vi "RT main.vi"   [LabVIEW 2015]
uses:
  Setpoints.ctl
  <vilib>/Utility/error.llb/Error Cluster From Error Code.vi
  <vilib>/rvi/errors/niLvFpgaAdjustHostInterfaceError.vi
  <vilib>/FPGAPlugInAG/Dynamic/niLvFpga_Close_Dynamic.vi
  <vilib>/FPGAPlugInAG/cRIO-9118/niLvFpga_Open_cRIO-9118.vi
  <vilib>/rvi/interface/common/dynamic/niFpgaDynamicAddResources.vi
  <vilib>/FPGAPlugInAG/Dynamic/niLvFpga_Run_Dynamic.vi
  <vilib>/rvi/interface/nirviReadWriteControl/nirviReadWriteControl.xnode
  <vilib>/rvi/interface/nirviCloseFPGA/nirviCloseFPGA.xnode
  <vilib>/rvi/interface/nirviOpenFPGA/nirviOpenFPGA.xnode
  FPGA Bitfiles/TanqueQuadruplo_FPGATarget_FPGAmain_2eouoVfTWZU.lvbitx
  FPGA main.vi
  <vilib>/rvi/interface/nirviMethod/nirviMethod.xnode
  NiFpgaLv.dll
  <vilib>/rvi/interface/Simulation/niFpgaSimulationCallBeginRW.vi
types:
  T1 = typedef "Setpoints.ctl" = cluster{"Bomba 1":fxp<+/-,20,5>, "Bomba 2":fxp<+/-,20,5>, "Solenoide 1":bool, "Solenoide 2":bool, "Solenoide 3":bool, "Solenoide 4":bool, "Valvula proporcional 2":fxp<+/-,20,5>, "Valvula proporcional 1":fxp<+/-,20,5>}
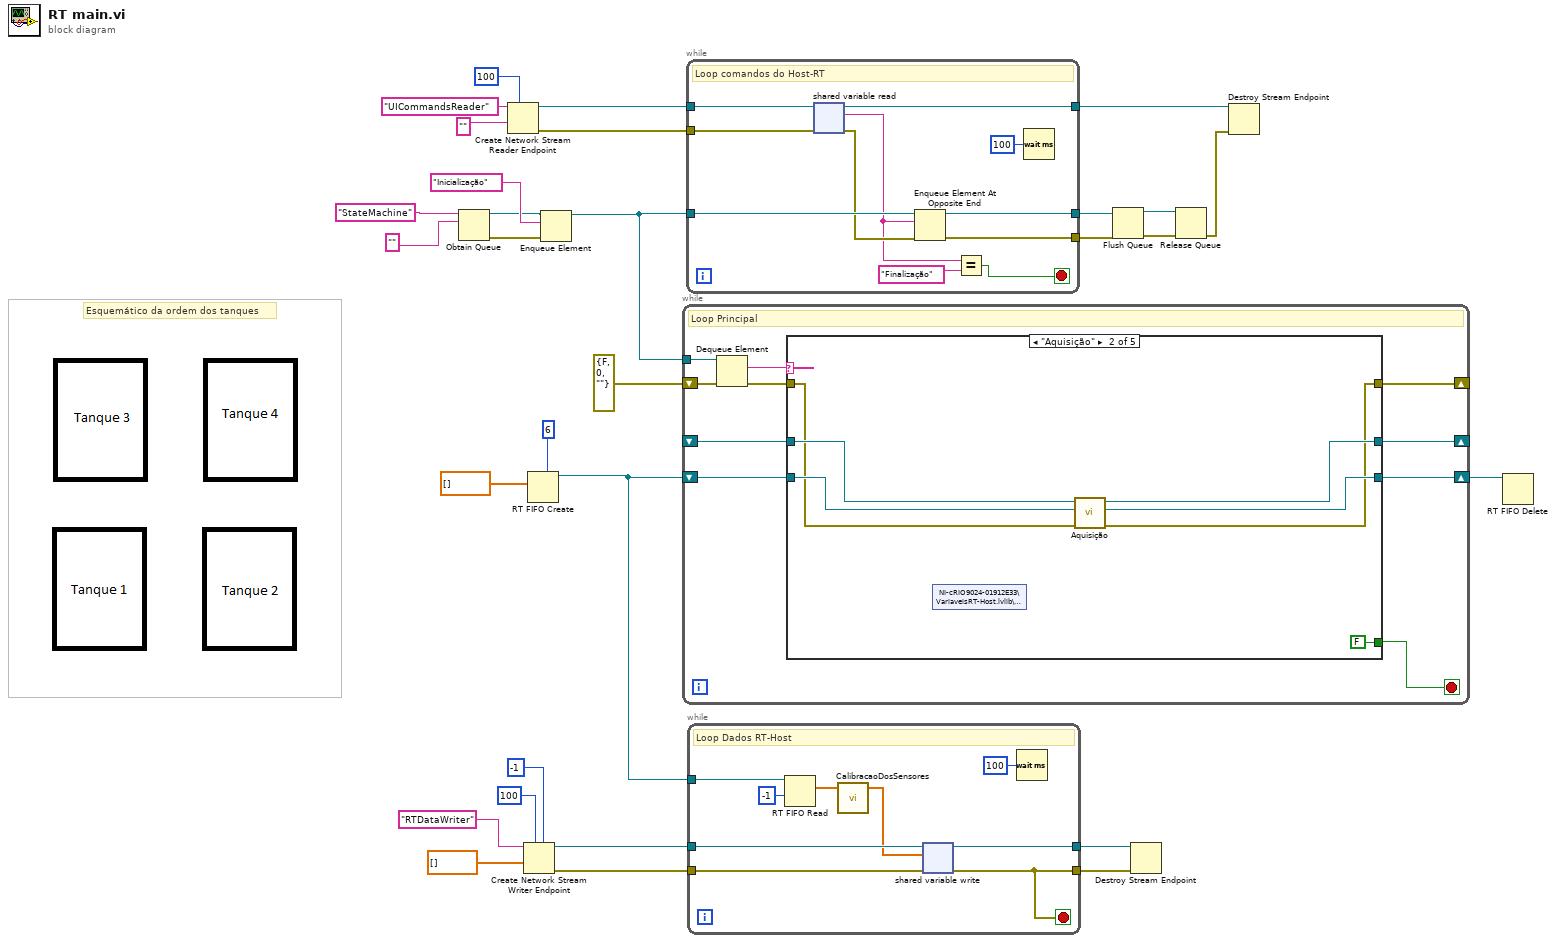
[diagram p0: block diagram]
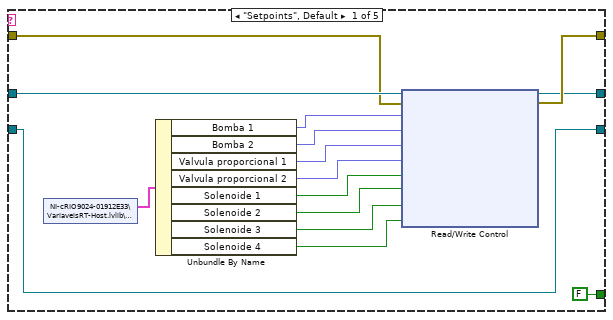
[diagram p2: hidden frame]
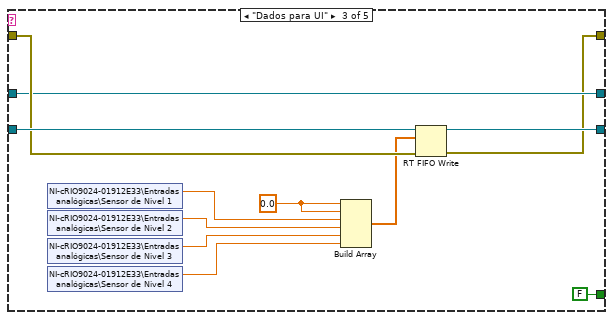
[diagram p3: hidden frame]
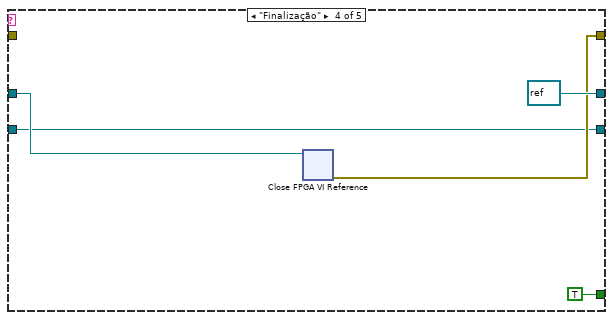
[diagram p4: hidden frame]
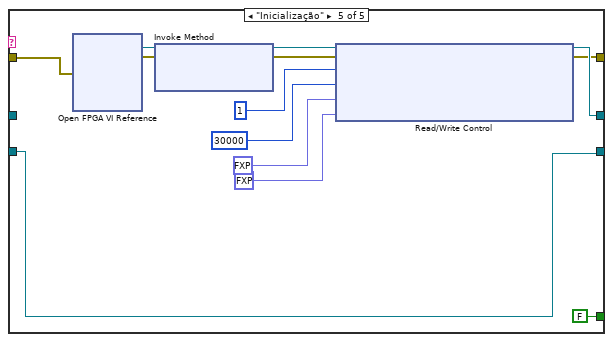
[diagram p5: hidden frame]
diagram:
  # "Esquemático da ordem dos tanques"
  n1 = Obtain Queue(name (unnamed)="StateMachine", element data type="") -> (queue out=w24:refnum<queue>, error out=w26:errorcluster)  [unwired: 3 in, 1 out]
  n2 = Create Network Stream Reader Endpoint(7:100 ("reader buffer size"), 9:"", 11:"UICommandsReader" ("reader name")) -> (0:w5:errorcluster, 3:w30:refnum<k21>)  [unwired: 4 in]
  n3 = Create Network Stream Writer Endpoint(5:-1 ("timeout in ms (-1)"), 7:100 ("writer buffer size"), 9:dbl[] [] ("appended array"), 11:"RTDataWriter" ("writer name")) -> (0:w12:errorcluster, 3:w11:refnum<k21>)  [unwired: 3 in]
  n4 = RT FIFO Create(1:dbl[] [] ("appended array"), 6:u32 6 ("elements in array (1)")) -> (8:w10:refnum<k33>)  [unwired: 6 in, 2 out]
  n5 = Enqueue Element(queue=w24, element="Inicialização", error in (no error)=w26) -> (queue out=w17:refnum<queue>)  [unwired: 1 in, 2 out]
  n6 = while {
    tunnel: w17 -> [w40]
    shift-right: [w37] -> _
    shift-left: _ -> [w38]
    shift-right: [w34] -> w6
    shift-left: w10 -> [w35]
    shift-right: [w32] -> _
    shift-left: errorcluster {"status"=FALSE, "code"=0, "source"=""} ("error out") -> [w33]
    stop <- w31 stop-if-true
    # "Loop Principal"
    n7 = Dequeue Element(queue=w40, error in (no error)=w33) -> (element=w39:string, error out=w36:errorcluster)  [unwired: 1 in, 2 out]
    n8 = case shown="\"Aquisição\"" w39 {
      tunnel: [w46 w57 w64 w77 w83] -> w32
      tunnel: w38 -> [w45 w62 w65 w79 _]
      tunnel: [w44 w61 w65 refnum<k20> refnum ("FPGA VI Reference Out") w86] -> w37
      tunnel: w36 -> [w42 w58 w73 _ w85]
      tunnel: w35 -> [w43 w60 w74 w76 w84]
      tunnel: [w43 w59 w66 w76 w84] -> w34
      tunnel: [FALSE FALSE FALSE TRUE FALSE] -> w31
      frame "Setpoints", Default {
        n9 = shared-variable "NI-cRIO9024-01912E33\\VariaveisRT-Host.lvlib\\Setpoints"() -> (w55:T1)  [unwired: 1 in, 1 out]
        n10 = Unbundle By Name(w55) -> ("Bomba 1"=w54:fxp<+/-,20,5>, "Bomba 2"=w53:fxp<+/-,20,5>, "Valvula proporcional 1"=w52:fxp<+/-,20,5>, "Valvula proporcional 2"=w51:fxp<+/-,20,5>, "Solenoide 1"=w50:bool, "Solenoide 2"=w49:bool, "Solenoide 3"=w48:bool, "Solenoide 4"=w47:bool)
        n11 = xnode "Read/Write Control"("FPGA VI Reference In"=w45, "error in"=w42, "Bomba 1"=w54, "Bomba 2"=w53, "Valvula proporcional 1"=w52, "Valvula proporcional 2"=w51, "Solenoide 1"=w50, "Solenoide 2"=w49, "Solenoide 3"=w48, "Solenoide 4"=w47) -> ("FPGA VI Reference Out"=w44:refnum<k20>, "error out"=w46:errorcluster)
      }
      frame "Aquisição" {
        n12 = shared-variable "NI-cRIO9024-01912E33\\VariaveisRT-Host.lvlib\\Setpoints"() -> ()  [unwired: 1 in, 2 out]
        n13 = call "Aquisição.vi"("error in (no error)"=w58, "rt fifo"=w60, "FPGA VI Reference In"=w62) -> ("error out"=w57:errorcluster, "rt fifo 2"=w59:refnum<k33>, "FPGA VI Reference Out"=w61:refnum<k20>)  [unwired: 6 in]
      }
      frame "Dados para UI" {
        w68 = 0.0
        n14 = shared-variable "NI-cRIO9024-01912E33\\Entradas analógicas\\Sensor de Nivel 1"() -> (w69:dbl)  [unwired: 1 in, 1 out]
        n15 = shared-variable "NI-cRIO9024-01912E33\\Entradas analógicas\\Sensor de Nivel 2"() -> (w70:dbl)  [unwired: 1 in, 1 out]
        n16 = shared-variable "NI-cRIO9024-01912E33\\Entradas analógicas\\Sensor de Nivel 3"() -> (w71:dbl)  [unwired: 1 in, 1 out]
        n17 = shared-variable "NI-cRIO9024-01912E33\\Entradas analógicas\\Sensor de Nivel 4"() -> (w72:dbl)  [unwired: 1 in, 1 out]
        n18 = Build Array(w68, w68, w69, w70, w71, w72) -> (w67:dbl[])
        n19 = RT FIFO Write(0:w74, 1:w67, 3:w73) -> (8:w66:refnum<k33>, 11:w64:errorcluster)  [unwired: 2 in, 2 out]
      }
      frame "Finalização" {
        n20 = xnode "Close FPGA VI Reference"("FPGA VI Reference In"=w79) -> ("error out"=w77:errorcluster)  [unwired: 1 in]
      }
      frame "Inicialização" {
        n21 = xnode "Open FPGA VI Reference"("error in"=w85) -> ("FPGA VI Reference Out"=w92:refnum<k20>, "error out"=w91:errorcluster)  [unwired: 1 in]
        n22 = xnode "Invoke Method"("FPGA VI Reference In"=w92, "error in"=w91) -> ("FPGA VI Reference Out"=w90:refnum<k20>, "error out"=w89:errorcluster)  [unwired: 1 in]
        n23 = xnode "Read/Write Control"("FPGA VI Reference In"=w90, "error in"=w89, "Temporização FPGA"=u32 1, "Tempo de despejo de emergência (mSec)"=u32 30000, "Bomba 1"=fxp<+/-,20,5> 0.0, "Bomba 2"=fxp<+/-,20,5> 0.0) -> ("FPGA VI Reference Out"=w86:refnum<k20>, "error out"=w83:errorcluster)
      }
    }
  }
  n24 = while {
    tunnel: w30 -> [w103]
    tunnel: [w102] -> w29
    tunnel: w5 -> [w101]
    tunnel: w17 -> [w100]
    tunnel: [w99] -> w8
    tunnel: [w97] -> w9
    stop <- w94 stop-if-true
    # "Loop comandos do Host-RT"
    n25 = shared-variable-read(w103, w101) -> (w102:refnum<k21>, w98:errorcluster, w96:string)  [unwired: 1 in, 1 out]
    n26 = Enqueue Element At Opposite End(queue=w100, element=w96, error in (no error)=w98) -> (queue out=w99:refnum<queue>, error out=w97:errorcluster)  [unwired: 1 in, 1 out]
    n27 = Equal?(x=w96, y="Finalização") -> (x = y?=w94:bool)
    n28 = Wait (ms)(milliseconds to wait=u32 100) -> ()  [unwired: 1 out]
  }
  n29 = while {
    tunnel: w10 -> [w112]
    tunnel: w11 -> [w111]
    tunnel: w12 -> [w110]
    tunnel: [w109] -> w13
    tunnel: [w107] -> w14
    stop <- w107 stop-if-true
    # "Loop Dados RT-Host"
    n30 = RT FIFO Read(0:w112, 2:-1 ("timeout in ms (0)")) -> (9:w105:dbl[])  [unwired: 2 in, 4 out]
    n31 = call "CalibracaoDosSensores.vi"("Pump and sensor data in"=w105) -> ("Pump and sensor data out"=w104:dbl[])  [unwired: 4 in]
    n32 = shared-variable-write(w111, w110, w104) -> (w109:refnum<k21>, w107:errorcluster)  [unwired: 1 in, 1 out]
    n33 = Wait (ms)(milliseconds to wait=u32 100) -> ()  [unwired: 1 out]
  }
  n34 = Flush Queue(queue=w8, error in (no error)=w9) -> (queue out=w21:refnum<queue>, error out=w20:errorcluster)  [unwired: 1 out]
  n35 = Destroy Stream Endpoint(8:w14, 11:w13) -> ()  [unwired: 1 out]
  n36 = Release Queue(queue=w21, error in (no error)=w20) -> (error out=w7:errorcluster)  [unwired: 1 in, 2 out]
  n37 = Destroy Stream Endpoint(8:w7, 11:w29) -> ()  [unwired: 1 out]
  n38 = RT FIFO Delete(0:w6) -> ()  [unwired: 2 in, 1 out]
